vi "torque_and_rpm.vi"(6 "rpm_voltage":dbl, 8 "rpm_offszet":dbl, 9 "tq_offszet":dbl, 10 "tq_voltage":dbl, 11 "offset":bool) -> (1 "tq":dbl, 2 "rpm_offset":dbl, 3 "tq_offset":dbl, 4 "rpm":dbl)   [LabVIEW 2014]
uses:
  <vilib>/ptbypt/NI_PtbyPt.lvlib
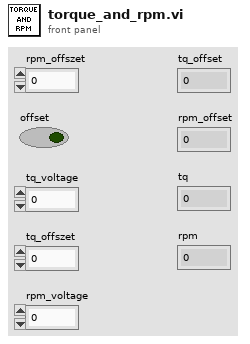
[diagram p1: front panel]
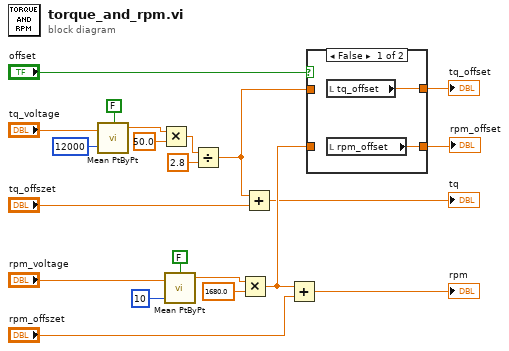
[diagram p0: block diagram]
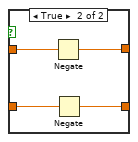
[diagram p2: hidden frame]
diagram:
  n1 = call <vilib>:"Mean PtByPt.vi"("x"="tq_voltage", "sample length"=12000, "initialize"=FALSE) -> ("mean"=w18:dbl)  [unwired: 1 in, 1 out]
  n2 = Multiply(x=w18, y=50.0) -> (x*y=w14:dbl)
  n3 = call <vilib>:"Mean PtByPt.vi"("x"="rpm_voltage", "sample length"=10, "initialize"=FALSE) -> ("mean"=w9:dbl)  [unwired: 1 in, 1 out]
  n4 = Divide(x=w14, y=2.8) -> (x/y=w15:dbl)
  n5 = Multiply(x=w9, y=1680.0) -> (x*y=w16:dbl)
  n6 = Add(x=w15, y="tq_offszet") -> (x+y=→"tq":dbl)
  n7 = Add(x=w16, y="rpm_offszet") -> (x+y=→"rpm":dbl)
  n8 = case shown="False" "offset" {
    tunnel: w15 -> [_ w27]
    tunnel: w16 -> [_ w26]
    tunnel: [w23 w25] -> w20
    tunnel: [w22 w24] -> w21
    frame False {
      n9 = local read "tq_offset"() -> (w23:dbl)
      n10 = local read "rpm_offset"() -> (w22:dbl)
    }
    frame True {
      n11 = Negate(x=w27) -> (-x=w25:dbl)
      n12 = Negate(x=w26) -> (-x=w24:dbl)
    }
  }
  "rpm_offset" <- w21
  "tq_offset" <- w20
